vi "Set Value Options.vi"(7 "type":variant, 8 "error in (no error)":errorcluster, 9 "set default values":bool, 10 "populate values":bool, 11 "Control in":refnum<vi>) -> (0 "error out":errorcluster, 3 "Control out":refnum<vi>)   [LabVIEW 2017, in "Advanced Variant Tools.lvlib" / "Control Scripting.lvlib"]
uses:
  Control Scripting.lvlib
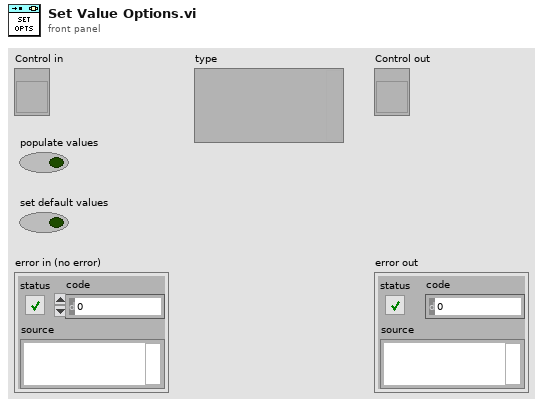
[diagram p1: front panel]
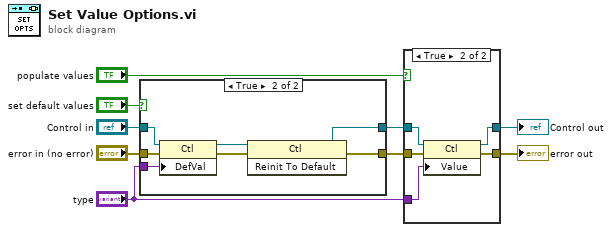
[diagram p0: block diagram]
diagram:
  n1 = case shown="True" "set default values" {
    tunnel: "error in (no error)" -> [w10 w18]
    tunnel: [w10 w14] -> w5
    tunnel: [w11 w12] -> w4
    tunnel: "Control in" -> [w11 w16]
    tunnel: "type" -> [_ w15]
    frame False {
    }
    frame True {
      n2 = property class="Ctl"(reference=w16, error in=w18, "DefVal"=w15) -> (reference out=w13:refnum<vi>, error out=w17:errorcluster)
      n3 = invoke class="Ctl" method="Reinit To Default"(reference=w13, error in=w17) -> (reference out=w12:refnum<vi>, error out=w14:errorcluster)  [unwired: 1 in, 1 out]
    }
  }
  n4 = case shown="True" "populate values" {
    tunnel: w5 -> [w19 w25]
    tunnel: [w19 w24] -> w8
    tunnel: [w20 w23] -> w9
    tunnel: w4 -> [w20 w22]
    tunnel: "type" -> [_ w21]
    frame False {
    }
    frame True {
      n5 = property class="Ctl"(reference=w22, error in=w25, "Value"=w21) -> (reference out=w23:refnum<vi>, error out=w24:errorcluster)
    }
  }
  "Control out" <- w9
  "error out" <- w8
